vi "创建数据库表.vi"() -> ()   [LabVIEW 2018]
panel:
  out "连接的字符串":string
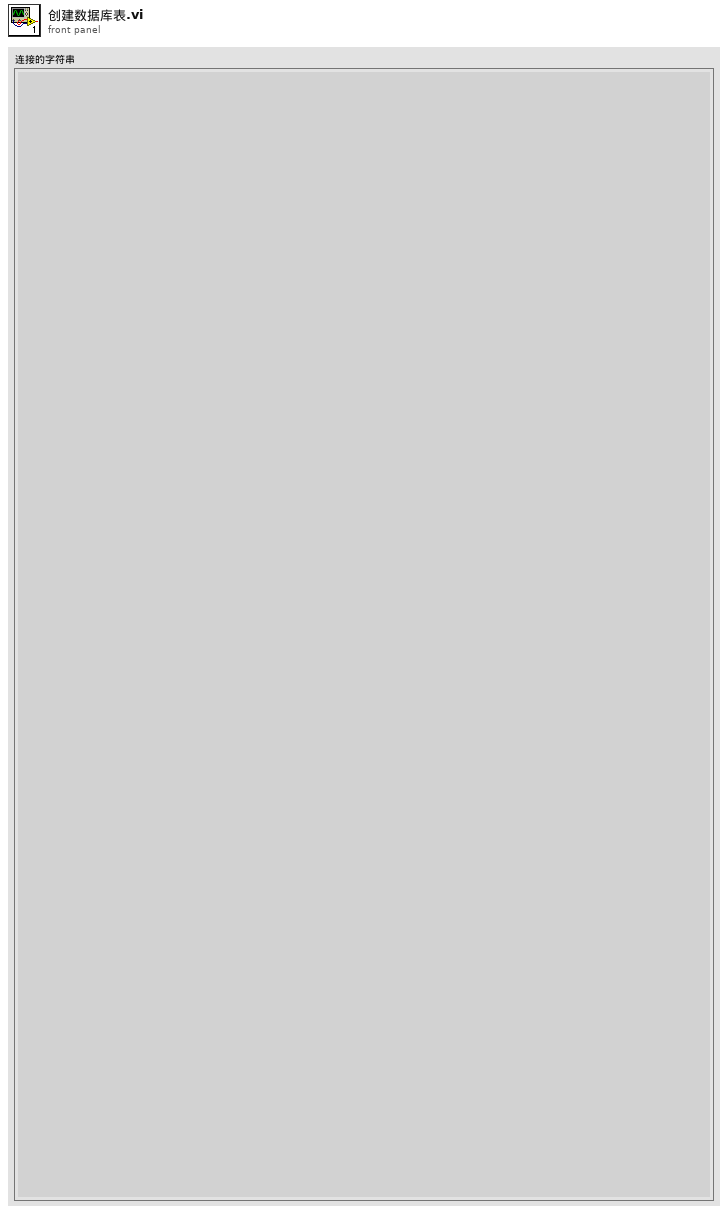
[diagram p1: front panel]
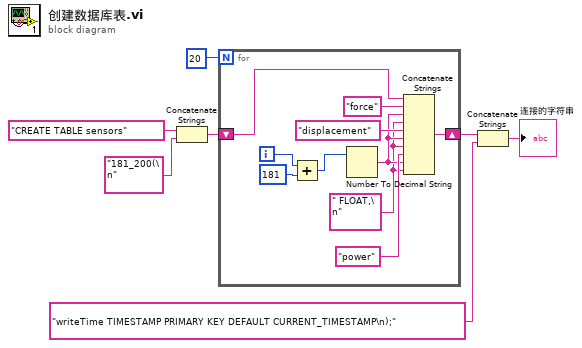
[diagram p0: block diagram]
diagram:
  n1 = Concatenate Strings("CREATE TABLE sensors", "181_200(\n") -> (w5:string)
  n2 = for {
    N: 20 -> [_]
    shift-right: [w16] -> w3
    shift-left: w5 -> [w17]
    i -> [w14]
    w8 = " FLOAT,\n" ("字符串")
    n3 = Add(x=w14, y=181) -> (x+y=w12:i32)
    n4 = Number To Decimal String(number=w12) -> (decimal integer string=w9:string)  [unwired: 1 in]
    n5 = Concatenate Strings(w17, "force" ("字符串"), w9, w8, "displacement" ("字符串"), w9, w8, "power" ("字符串"), w9, w8) -> (w16:string)
  }
  n6 = Concatenate Strings(w3, "writeTime TIMESTAMP PRIMARY KEY DEFAULT CURRENT_TIMESTAMP\n);" ("字符串")) -> (→"连接的字符串":string)
